vi "Write Loop.vi"(11 "Telemetry Server in":refnum<class "Telemetry Server.lvclass">) -> (3 "Telemetry Server out":refnum<class "Telemetry Server.lvclass">)   [LabVIEW 2020, in "VolatusTelemetry.lvlib" / "Telemetry Server.lvclass"]
uses:
  Telemetry Server.lvclass
  Telemetry Server.lvclass/Telemetry Server.ctl
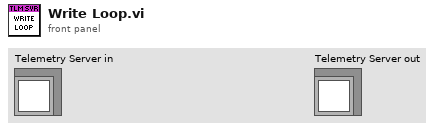
[diagram p1: front panel]
types:
  T1 = typedef "VolatusTelemetry.lvlib/Telemetry Server.lvclass/IPv4 Endpoint.ctl" = cluster{"Address":u32, "Port":u16}
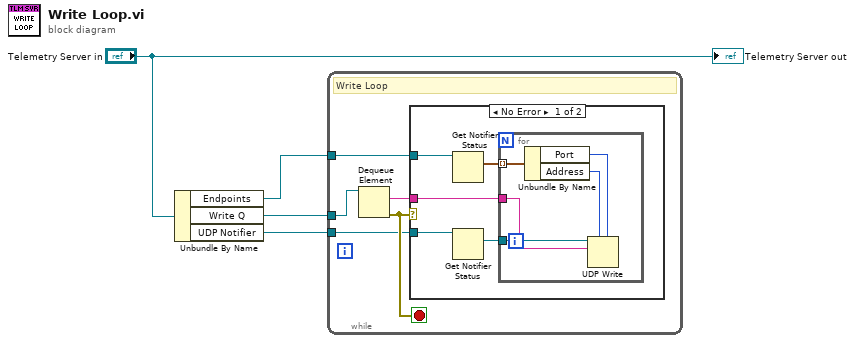
[diagram p0: block diagram]
diagram:
  n1 = Unbundle By Name("Telemetry Server in") -> ("Endpoints"=w2:refnum<notifier>, "Write Q"=w3:refnum<queue>, "UDP Notifier"=w4:refnum<notifier>)
  n2 = while {
    tunnel: w3 -> [w8]
    tunnel: w4 -> [w6]
    tunnel: w2 -> [w5]
    stop <- w9 stop-if-true
    # "Write Loop"
    n3 = Dequeue Element(queue=w8) -> (element=w7:string, error out=w9:errorcluster)  [unwired: 2 in, 2 out]
    n4 = case shown="No Error" w9 {
      tunnel: w7 -> [w10 _]
      tunnel: w6 -> [w14 _]
      tunnel: w5 -> [w12 _]
      frame No Error {
        n5 = Get Notifier Status(notifier=w12) -> (current notification=w11:T1[])  [unwired: 1 in, 4 out]
        n6 = Get Notifier Status(notifier=w14) -> (current notification=w13:refnum<k16>)  [unwired: 1 in, 4 out]
        n7 = for {
          tunnel: w13 -> [w19]
          tunnel: w11 -> [w16] mode=indexing
          tunnel: w10 -> [w15]
          n8 = Unbundle By Name(w16) -> ("Port"=w17:u16, "Address"=w18:u32)
          n9 = UDP Write(address=w18, port or service name=w17, connection ID=w19, data in=w15) -> ()  [unwired: 2 in, 2 out]
        }
      }
      frame Error {
      }
    }
  }
  "Telemetry Server out" <- "Telemetry Server in"
